vi "SubscriberDataFGV.vi"(0 "variable":string, 1 "command":T3, 5 "variable type":string, 7 "connection ID":refnum<k5>, 9 "local":bool=TRUE, 11 "error in (no error)":errorcluster, 12 "spawn":bool=TRUE) -> (4 "variable data":T2, 6 "all variables":string[](array[string]), 8 "connection data":T1, 10 "all connections":refnum<k5>[](array[refnum]), 15 "error out":errorcluster)   [LabVIEW 2011]
uses:
  FGV_Control.ctl
  variabledata_typdef.ctl
  connectiondata_typdef.ctl
panel:
  out "variable variant out":variant
  out "Variant Out":variant
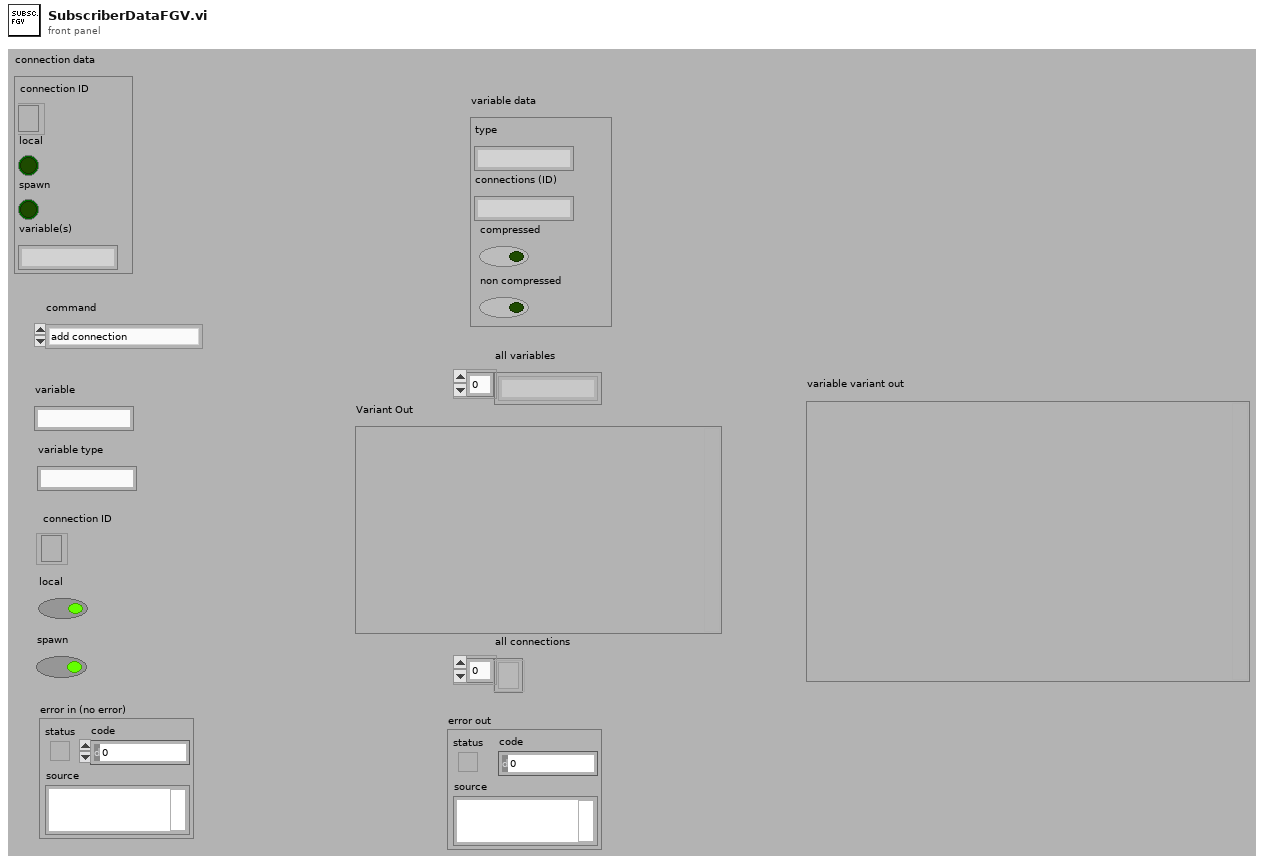
[diagram p1: front panel]
types:
  T1 = typedef "connectiondata_typdef.ctl" = cluster{"connection ID":refnum<k5>, "local":bool, "spawn":bool, "variable(s)":string}
  T2 = typedef "variabledata_typdef.ctl" = cluster{"type":string, "connections (ID)":string, "compressed":bool, "non compressed":bool}
  T3 = typedef "FGV_Control.ctl" = enum16{"add connection", "remove connection", "read variable data", "read connection data", "return all connections", "return all variables", "reset"}
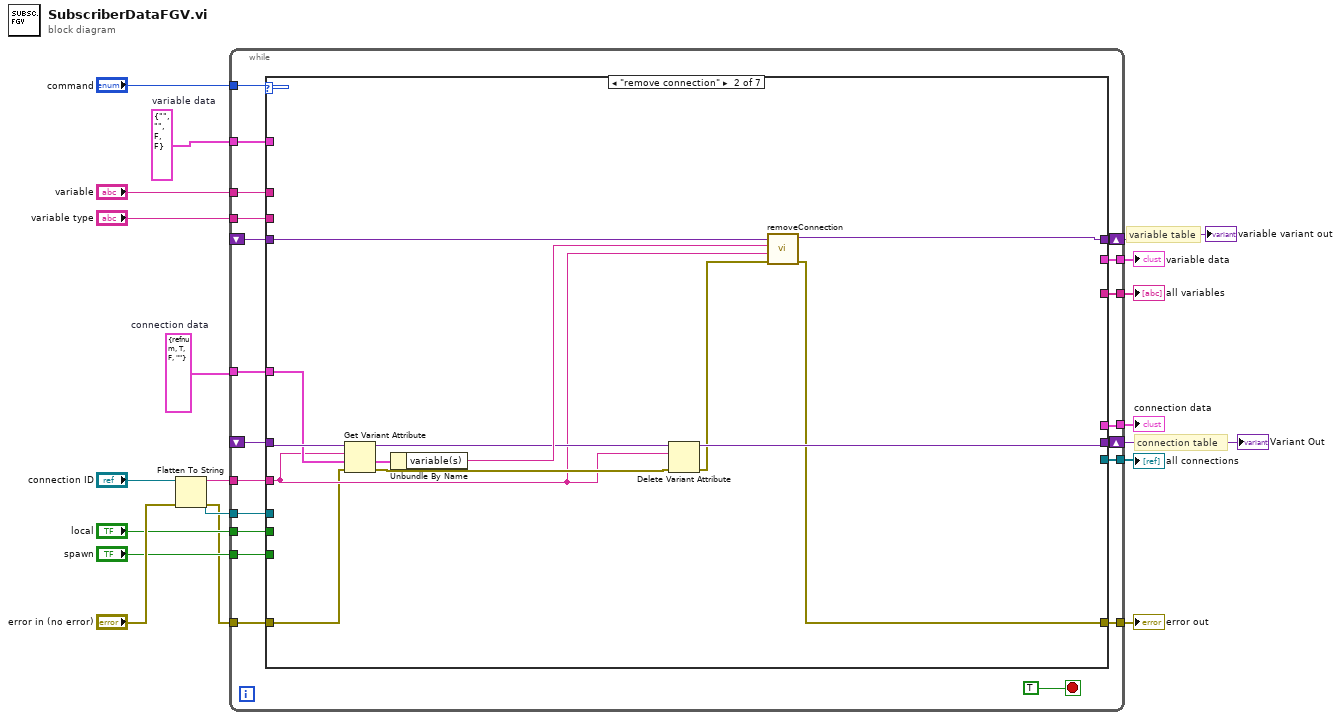
[diagram p0: block diagram]
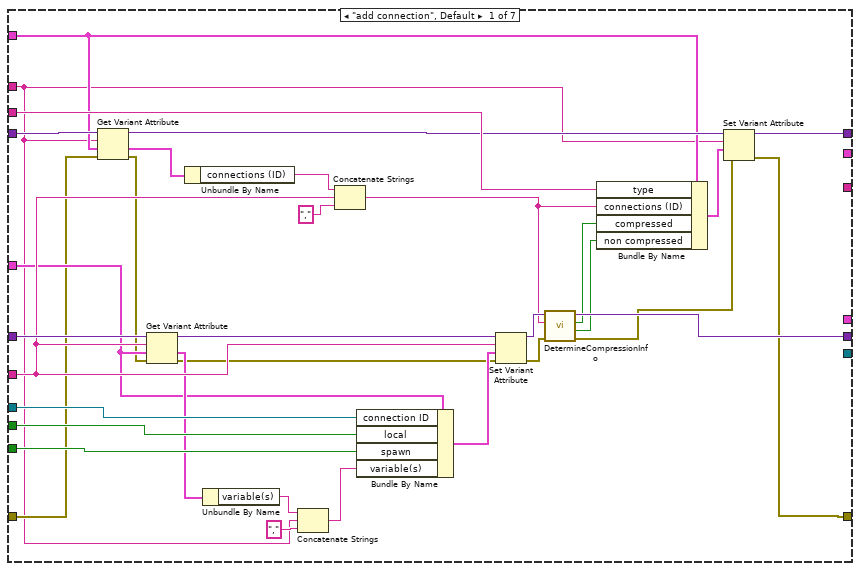
[diagram p2: hidden frame]
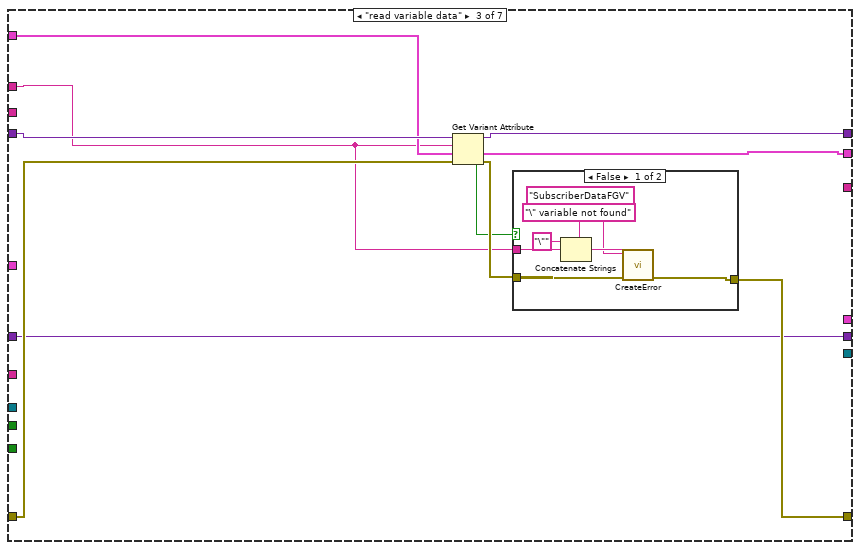
[diagram p3: hidden frame]
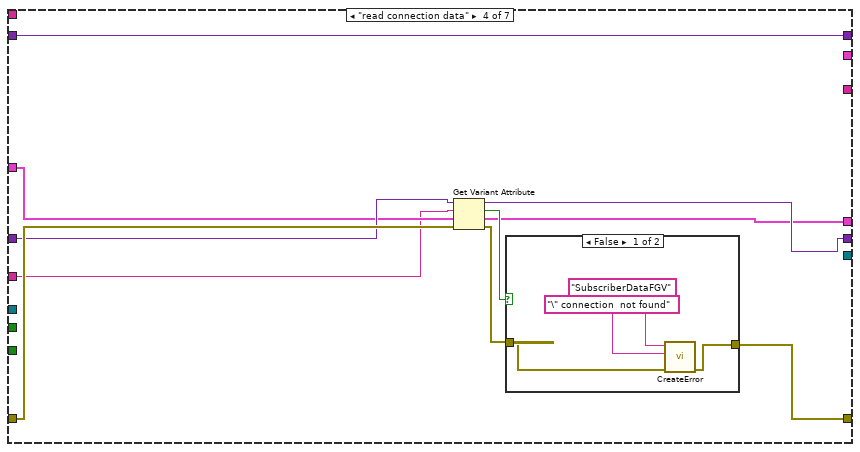
[diagram p5: hidden frame]
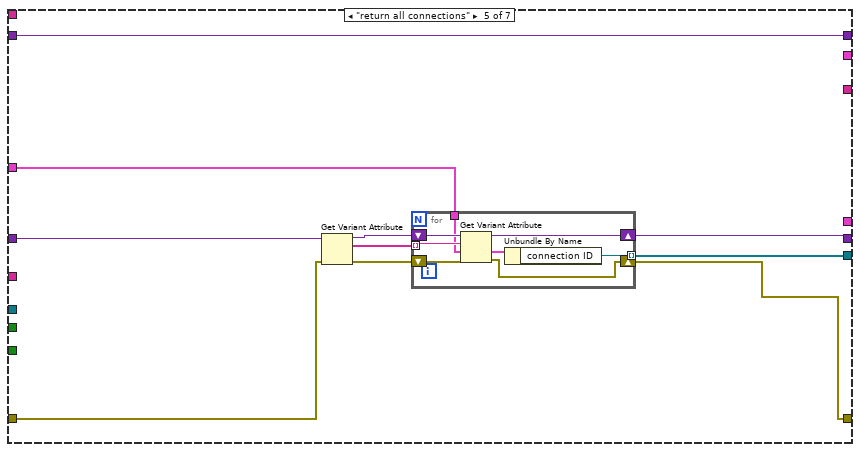
[diagram p7: hidden frame]
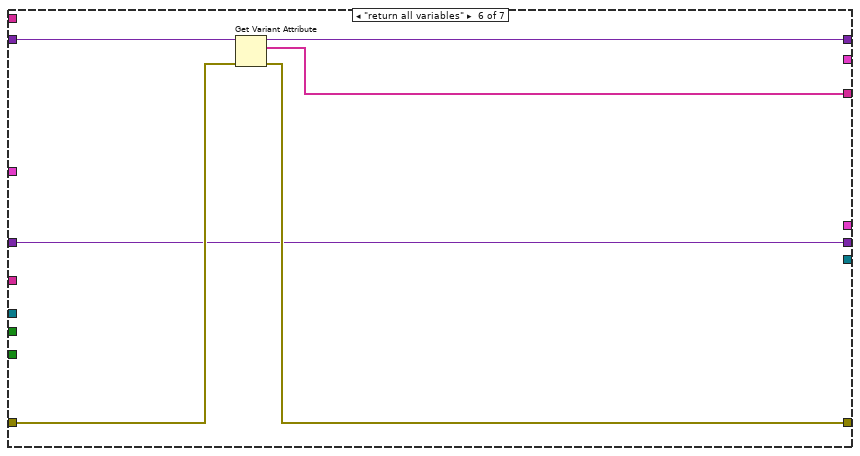
[diagram p8: hidden frame]
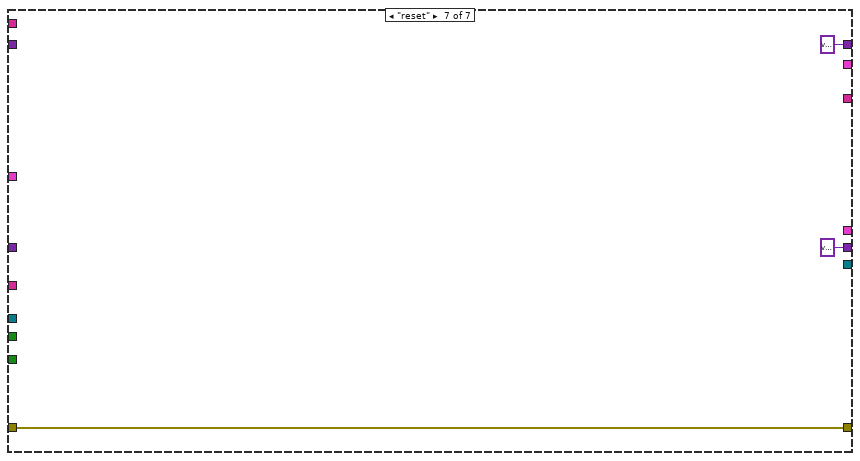
[diagram p9: hidden frame]
diagram:
  w9 = T2 {"type"="", "connections (ID)"="", "compressed"=FALSE, "non compressed"=FALSE}  # variable data
  w10 = T1 {"connection ID"=refnum, "local"=TRUE, "spawn"=FALSE, "variable(s)"=""}  # connection data
  # "connection table"
  # "variable table"
  n1 = Flatten To String(anything="connection ID", error in (no error)="error in (no error)") -> (data string=w14:string, error out=w7:errorcluster)  [unwired: 2 in, 1 out]
  n2 = while {
    shift-right: [w38] -> w1
    shift-left: _ -> [w27]
    shift-right: [w37] -> w2
    shift-left: _ -> [w33]
    tunnel: "command" -> [w35]
    tunnel: "variable type" -> [w34]
    tunnel: "variable" -> [w32]
    tunnel: w14 -> [w31]
    tunnel: "connection ID" -> [w30]
    tunnel: "local" -> [w29]
    tunnel: "spawn" -> [w28]
    tunnel: w10 -> [w26]
    tunnel: w9 -> [w25]
    tunnel: [w24] -> w8
    tunnel: w7 -> [w23]
    tunnel: [w22] -> w6
    tunnel: [w21] -> w5
    tunnel: [w20] -> w4
    tunnel: [w19] -> w3
    stop <- TRUE stop-if-true
    n3 = case shown="\"remove connection\"" w35 {
      tunnel: [w47 w80 w93 w103 w118 w140 variant ("variable variant out")] -> w38
      tunnel: [w60 w75 w87 w107 w124 w136 variant ("Variant Out")] -> w37
      tunnel: w34 -> [w71 _ _ _ _ _ _]
      tunnel: w33 -> [w58 w84 w87 w108 w127 w136 _]
      tunnel: w32 -> [w39 _ w85 _ _ _ _]
      tunnel: w31 -> [w56 w76 _ w105 _ _ _]
      tunnel: w30 -> [w68 _ _ _ _ _ _]
      tunnel: w29 -> [w67 _ _ _ _ _ _]
      tunnel: w28 -> [w66 _ _ _ _ _ _]
      tunnel: w27 -> [w65 w81 w94 w103 w118 w141 _]
      tunnel: w26 -> [w46 w83 _ w106 w123 _ _]
      tunnel: w25 -> [w45 _ w92 _ _ _ _]
      tunnel: [_ _ w88 _ _ _ _] -> w24
      tunnel: w23 -> [w43 w74 w90 w110 w121 w138 w142]
      tunnel: [w40 w72 w89 w109 w119 w137 w142] -> w22
      tunnel: [_ _ _ w104 _ _ _] -> w21
      tunnel: [_ _ _ _ w122 _ _] -> w20
      tunnel: [_ _ _ _ _ w139 _] -> w19
      frame "add connection", Default {
        n4 = Get Variant Attribute(Variant=w65, name=w39, default value (empty Variant)=w45, error in=w43) -> (duplicate Variant=w64:variant, value=w63:T2, error out=w42:errorcluster)  [unwired: 1 out]
        n5 = Get Variant Attribute(Variant=w58, name=w56, default value (empty Variant)=w46, error in=w42) -> (duplicate Variant=w57:variant, value=w55:T1, error out=w44:errorcluster)  [unwired: 1 out]
        n6 = Unbundle By Name(w63) -> ("connections (ID)"=w59:string)
        n7 = Unbundle By Name(w55) -> ("variable(s)"=w53:string)
        n8 = Concatenate Strings(w53, w39, "," ("string")) -> (w48:string)
        n9 = Concatenate Strings(w59, w56, "," ("string")) -> (w52:string)
        n10 = Bundle By Name(cluster=w46, "connection ID"=w68, "local"=w67, "spawn"=w66, "variable(s)"=w48) -> (w69:T1)
        n11 = Set Variant Attribute(Variant=w57, name=w56, value=w69, error in=w44) -> (Variant out=w61:variant, error out=w51:errorcluster)  [unwired: 1 out]
        n12 = call "DetermineCompressionInfo.vi"("error in (no error)"=w51, "connections (ID)"=w52, "Variant In"=w61) -> ("error out"=w41:errorcluster, "non compressed"=w49:bool, "compressed"=w50:bool, "Variant Out"=w60:variant)  [unwired: 5 in]
        n13 = Bundle By Name(cluster=w45, "type"=w71, "connections (ID)"=w52, "compressed"=w50, "non compressed"=w49) -> (w70:T2)
        n14 = Set Variant Attribute(Variant=w64, name=w39, value=w70, error in=w41) -> (Variant out=w47:variant, error out=w40:errorcluster)  [unwired: 1 out]
      }
      frame "remove connection" {
        n15 = Get Variant Attribute(Variant=w84, name=w76, default value (empty Variant)=w83, error in=w74) -> (duplicate Variant=w78:variant, value=w82:T1, error out=w77:errorcluster)  [unwired: 1 out]
        n16 = Unbundle By Name(w82) -> ("variable(s)"=w79:string)
        n17 = Delete Variant Attribute(4:w77, 6:w76, 7:w78) -> (0:w73:errorcluster, 3:w75:variant)  [unwired: 1 out]
        n18 = call "removeConnection.vi"("error in (no error) 2"=w73, "conection id (string)"=w76, "variable(s)"=w79, "variable variant in"=w81) -> ("error out"=w72:errorcluster, "variable variant out"=w80:variant)  [unwired: 6 in]
      }
      frame "read variable data" {
        n19 = Get Variant Attribute(Variant=w94, name=w85, default value (empty Variant)=w92, error in=w90) -> (duplicate Variant=w93:variant, found=w86:bool, value=w88:T2, error out=w91:errorcluster)
        n20 = case shown="False" w86 {
          tunnel: w91 -> [w101 w102]
          tunnel: [w100 w102] -> w89
          tunnel: w85 -> [w98 _]
          frame False {
            n21 = Concatenate Strings("\"" ("string"), w98, "\" variable not found" ("error message (\"\")")) -> (w96:string)
            n22 = call "CreateError.vi"("user error in"=w101, "error message (\"\")"=w96, "command"="SubscriberDataFGV") -> ("user error  out"=w100:errorcluster)  [unwired: 8 in]
          }
          frame True {
          }
        }
      }
      frame "read connection data" {
        n23 = Get Variant Attribute(Variant=w108, name=w105, default value (empty Variant)=w106, error in=w110) -> (duplicate Variant=w107:variant, found=w112:bool, value=w104:T1, error out=w111:errorcluster)
        n24 = case shown="False" w112 {
          tunnel: w111 -> [w115 w117]
          tunnel: [w114 w117] -> w109
          frame False {
            n25 = call "CreateError.vi"("user error in"=w115, "error message (\"\")"="\" connection  not found" ("error message (\"\")"), "command"="SubscriberDataFGV") -> ("user error  out"=w114:errorcluster)  [unwired: 8 in]
          }
          frame True {
          }
        }
      }
      frame "return all connections" {
        n26 = Get Variant Attribute(Variant=w127, error in=w121) -> (duplicate Variant=w125:variant, names=w126:string[], error out=w120:errorcluster)  [unwired: 2 in, 1 out]
        n27 = for {
          tunnel: w126 -> [w133] mode=indexing
          tunnel: w123 -> [w131]
          tunnel: [w130] -> w122 mode=indexing
          shift-right: [w134] -> w124
          shift-left: w125 -> [w135]
          shift-right: [w128] -> w119
          shift-left: w120 -> [w129]
          n28 = Get Variant Attribute(Variant=w135, name=w133, default value (empty Variant)=w131, error in=w129) -> (duplicate Variant=w134:variant, value=w132:T1, error out=w128:errorcluster)  [unwired: 1 out]
          n29 = Unbundle By Name(w132) -> ("connection ID"=w130:refnum<k5>)
        }
      }
      frame "return all variables" {
        n30 = Get Variant Attribute(Variant=w141, error in=w138) -> (duplicate Variant=w140:variant, names=w139:string[], error out=w137:errorcluster)  [unwired: 2 in, 1 out]
      }
      frame "reset" {
      }
    }
  }
  "variable data" <- w8
  "error out" <- w6
  "connection data" <- w5
  "all connections" <- w4
  "all variables" <- w3
  "Variant Out" <- w2
  "variable variant out" <- w1
